vi "Read Error Count.vi"(11 "Test Case Result In":T1) -> (2 "Error count":i32, 3 "Test Case Result Out":T1)   [LabVIEW 2020, in "Test Case Result.lvlib"]
uses:
  Test Case Result.lvlib
  Test Case Result type.ctl
  Method Result/Method Result type.ctl
  Assertion Result/Public/TypeDefs/Status.ctl
  Assertion Result/Assertion Result type.ctl
  Assertion Result/Public/TypeDefs/Assertion Type.ctl
  Assertion Result/Assertion Result.lvlib
  Method Result/Method Result.lvlib
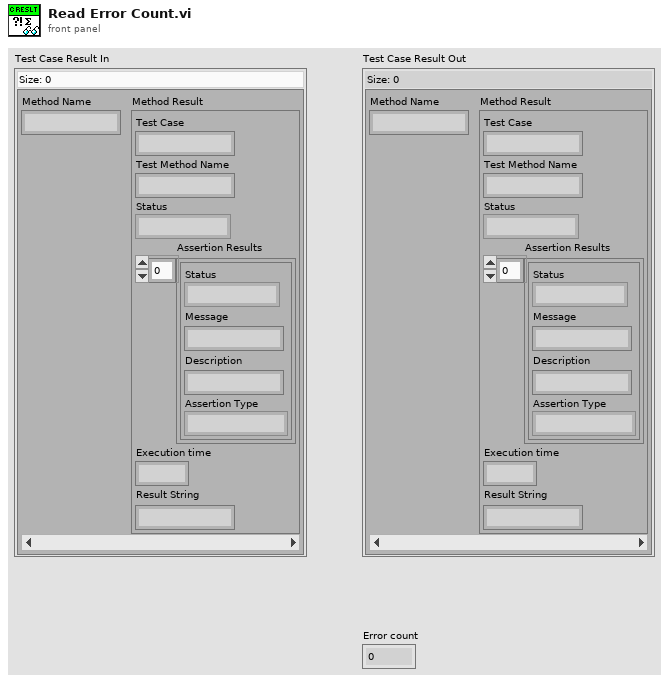
[diagram p1: front panel]
types:
  T1 = typedef "Test Case Result.lvlib/Test Case Result type.ctl" = map{string, T2}
  T2 = typedef "Method Result.lvlib/Method Result type.ctl" = cluster{"Test Case":string, "Test Method Name":string, "Status":T3, "Assertion Results":T4[], "Execution time":dbl, "Result String":string}
  T3 = typedef "Assertion Result.lvlib/Status.ctl" = enum16{"Pass", "Fail", "Error", "Skipped", "Setup Error", "Broken", "Teardown Error"}
  T4 = typedef "Assertion Result.lvlib/Assertion Result type.ctl" = cluster{"Status":T3, "Message":string, "Description":string, "Assertion Type":T5}
  T5 = typedef "Assertion Result.lvlib/Assertion Type.ctl" = enum16{"None", "Pass", "Fail", "Skip", "Pass if Equal", "Fail if Equal", "Pass if Error", "Fail if Error", "Pass if", "Fail if"}
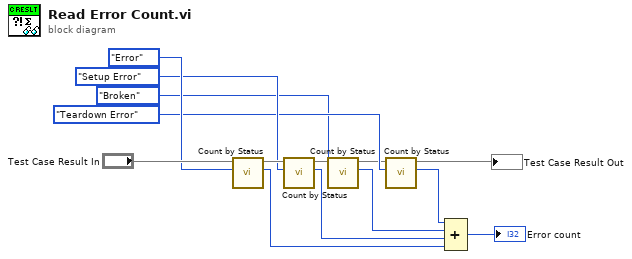
[diagram p0: block diagram]
diagram:
  n1 = call "Count by Status.vi"("Status"=Status."Error", "Test Case Result In"="Test Case Result In") -> ("Count"=w5:i32, "Test Case Result Out"=w13:T1)  [unwired: 8 in]
  n2 = call "Count by Status.vi"("Status"=Status."Setup Error", "Test Case Result In"=w13) -> ("Count"=w6:i32, "Test Case Result Out"=w4:T1)  [unwired: 8 in]
  n3 = call "Count by Status.vi"("Status"=Status."Broken", "Test Case Result In"=w4) -> ("Count"=w2:i32, "Test Case Result Out"=w3:T1)  [unwired: 8 in]
  n4 = call "Count by Status.vi"("Status"=Status."Teardown Error", "Test Case Result In"=w3) -> ("Count"=w7:i32, "Test Case Result Out"=→"Test Case Result Out":T1)  [unwired: 8 in]
  n5 = Compound Arithmetic op=ADD(w7, w2, w6, w5) -> (→"Error count":i32)
